vi "Initialize.vi"(11 "data in":refnum<class "EventMessengerMData.lvclass">) -> (1 "Event Registration Refnum":refnum<event-registration>, 3 "data out":refnum<class "EventMessengerMData.lvclass">)   [LabVIEW 2019, in "Event MessengerM.lvlib" / "EventMessengerMData.lvclass"]
uses:
  EventMessengerMData.lvclass
  EventMessengerMData.lvclass/EventMessengerMData.ctl
  Event Data.ctl
  Event MessengerM.lvlib
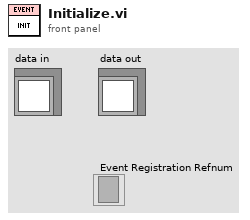
[diagram p1: front panel]
types:
  T1 = map{i32, cluster{"Write Count":u32, "Reg Refnum":u32, "aborted?":bool, "last element?":bool, "Event Refnum":refnum<user-event>}}
  T2 = cluster{"Write Count":u32, "Reg Refnum":u32, "aborted?":bool, "last element?":bool, "Event Refnum":refnum<user-event>}
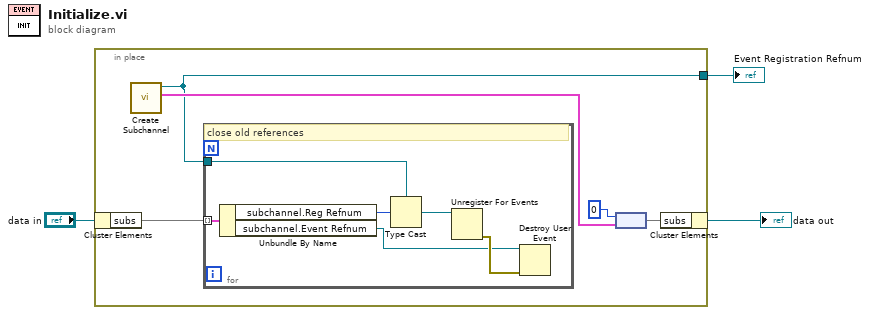
[diagram p0: block diagram]
diagram:
  n1 = in-place {
    in-place-border: [w6] -> w1
    n2 = in-place-cluster #1("data in") -> ("subs"=w8:T1)
    n3 = call "Create Subchannel.vi"() -> ("subchannel"=w7:T2, "Event Registration Refnum out"=w6:refnum<event-registration>)  [unwired: 10 in]
    n4 = for {
      tunnel: w8 -> [w11] mode=indexing
      tunnel: w6 -> [w14]
      # "close old references"
      n5 = Unbundle By Name(w11) -> ("subchannel.Reg Refnum"=w10:u32, "subchannel.Event Refnum"=w9:refnum<user-event>)
      n6 = Type Cast(type=w14, x=w10) -> (*(type *) &x=w13:refnum<event-registration>)
      n7 = Unregister For Events(event registration refnum=w13) -> (error out=w12:errorcluster)  [unwired: 1 in]
      n8 = Destroy User Event(user event=w9, error in=w12) -> ()  [unwired: 1 out]
    }
    n9 = node(0, w7) -> (w4:T1)
    n10 = in-place-cluster #1("subs"=w4) -> (→"data out":refnum<class "EventMessengerMData.lvclass">)
  }
  "Event Registration Refnum" <- w1
